vi "XYZ Ultrasonic Scanning Software 1.3.vi"() -> ()   [LabVIEW 2020]
doc: "The latest version of the ultrasonic scanning rig software."
uses:
  <instrlib>/Arcus Ethernet Driver 1.0.0/ArcusEthernetComm/classes/Controller/_Controller.lvclass
  <instrlib>/LeCroy Wave Series/LeCroy Wave Series.lvlib
panel:
  in  "stop":bool
  in  "Tab Control":T1(tab)
  in  "Check Osc Connection":bool
  out "Succesful Osc Connection":bool=TRUE
  in  "Check Rig Connection":bool
  out "Succesful Rig Connection":bool=TRUE
  in  "Error In":errorcluster
  in  "VISA Resource Name (Osc. Model Used)":refnum<visa-resource-name>
  in  "Move Y Distance":dbl
  in  "Set Starting Position":bool
  in  "Z Direction":bool=TRUE
  in  "Y Direction":bool=TRUE
  in  "Move X Distance":dbl
  in  "Move Z Distance":dbl
  in  "X Direction":bool=TRUE
  in  "Return To Home":bool
  in  "Move":bool
  in  "File Format":T2(radio)
  in  "File Name":string
  in  "Folder to Save A-Scan":path
  in  "Start A-Scan":bool
  in  "VISA resource name":refnum<visa-resource-name>
  in  "Source (0: Channel 1)":u16(ring) items=["Channel 1", "Channel 2", "Channel 3", "Channel 4", "Memory 1", "Memory 2", "Memory 3", "Memory 4", "Function 1", "Function 2", "Function 3", "Function 4", "Function 5", "Function 6", "Function 7", "Function 8"]
  out "A-Scan":waveform(dbl)(graph)
  in  "File Name for B-Scan":string
  in  "Folder to Save B-Scan":path
  in  "Folder to Save A-Scans":path
  in  "File Name for A-Scans":string
  in  "File Format":T2(radio)
  in  "Osc. Model":refnum<visa-resource-name>
  in  "Channel":u16(ring) items=["Channel 1", "Channel 2", "Channel 3", "Channel 4", "Memory 1", "Memory 2", "Memory 3", "Memory 4", "Function 1", "Function 2", "Function 3", "Function 4", "Function 5", "Function 6", "Function 7", "Function 8"]
  in  "Start B-Scan":bool
  in  "Initial X Direction":bool=TRUE
  in  "Initial Y Direction":bool=TRUE
  in  "Initial Z Direction":bool=TRUE
  in  "Confirm Scanning Parameters B-Scan":bool
  in  "Height (mm)":dbl
  in  "Width (mm)":dbl
  in  "Length (mm)":dbl
  in  "Select Axis To Scan":enum32{"No Selection", "X", "Y", "Z"}(radio)
  out "B-Scan":dbl[][](graph)
  in  "Folder to Save C-Scan":path
  in  "File Name for C-Scan":string
  in  "Source (0: Channel 1)":u16(ring) items=["Channel 1", "Channel 2", "Channel 3", "Channel 4", "Memory 1", "Memory 2", "Memory 3", "Memory 4", "Function 1", "Function 2", "Function 3", "Function 4", "Function 5", "Function 6", "Function 7", "Function 8"]
  in  "VISA resource name":refnum<visa-resource-name>
  in  "C-Scan Build Up Quantity":T3(radio)
  out "C-Scan":dbl[][](graph)
  in  "Scan C-Scan":bool
  in  "Length (mm)":dbl
  in  "Width (mm)":dbl
  in  "Height (mm)":dbl
  in  "?":bool
  in  "Initial X Direction":bool=TRUE
  in  "Initial Y Direction":bool=TRUE
  in  "Initial Z Direction":bool=TRUE
  in  "Select Plane To Scan":enum32{"No Selection", "XY", "XZ", "YZ"}(radio)
  in  "Folder to Save A-Scans":path
  in  "File Name for A-Scans":string
  in  "File Format":T2(radio)
  # "Moving To Starting Point (mm)"
  # "Scanning Tank Axes"
  # "Y"
  # "X"
  # "Z"
  # "Home ->"
  # "*Note - See user manual for scanning rig orientation to ensure correct axis directions"
  # "Scanning Parameters"
  # "Saving Parameters"
  # "Scanning Rig Parameters"
  # "Tank Dimensions"
  # "Y - Width"
  # "X - Length"
  # "Z - Height"
  # "Oscilloscope Parameters"
  # "Saving Parameters"
  # "*Note - See user manual for scanning rig orientation to ensure correct axis directions"
  # "Scanning Rig Parameters"
  # "Tank Dimensions"
  # "Y - Width"
  # "X - Length"
  # "Z - Height"
  # "Oscilloscope Parameters"
  # "Saving Parameters"
  # "*Note - See user manual for scanning rig orientation to ensure correct axis directions"
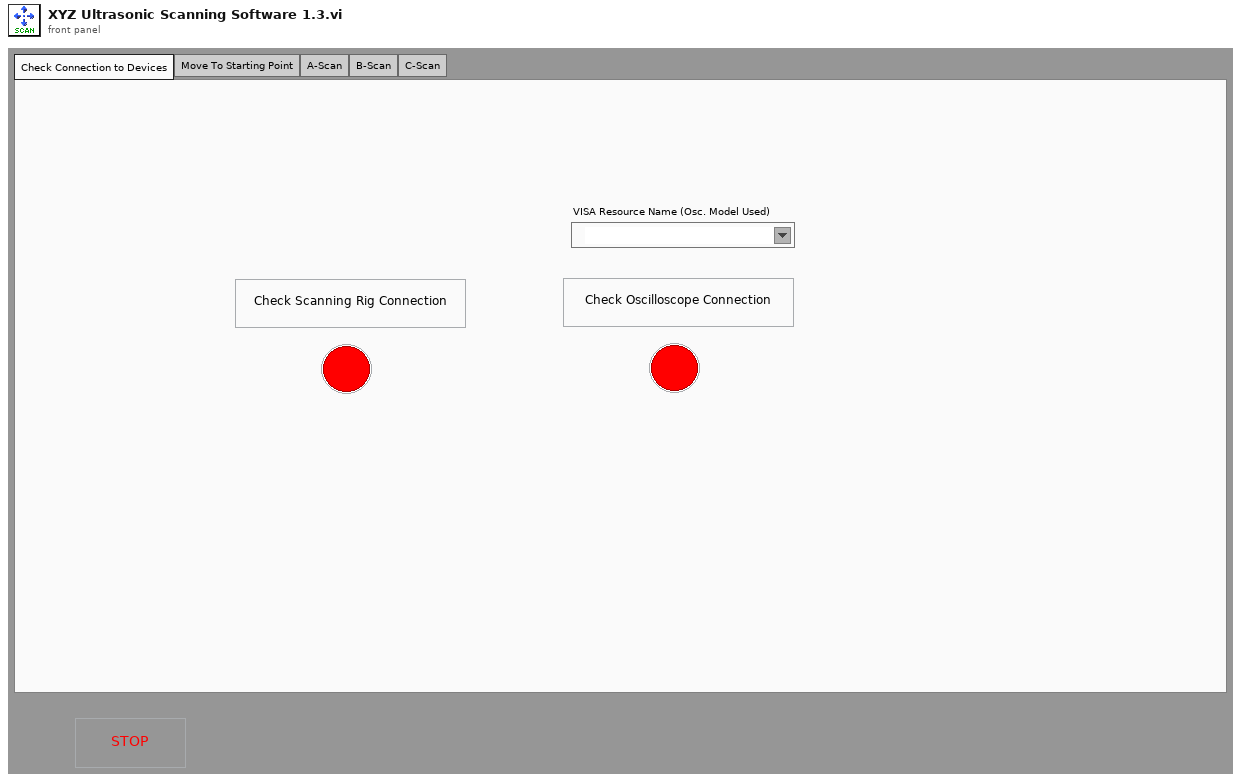
[diagram p1: front panel]
types:
  T1 = enum32{"Check Connection to Devices", "Move To Starting Point", "A-Scan", "B-Scan", "C-Scan"}
  T2 = enum32{"No Selection", "Do Not Save", "ASCII", "CSV", "MATLAB"}
  T3 = enum32{"No Selection", "Peak Positive", "Peak Negative", "Peak Magnitude", "Energy"}
  T4 = enum8{"Enabled", "Disabled", "Disabled and Grayed Out"}
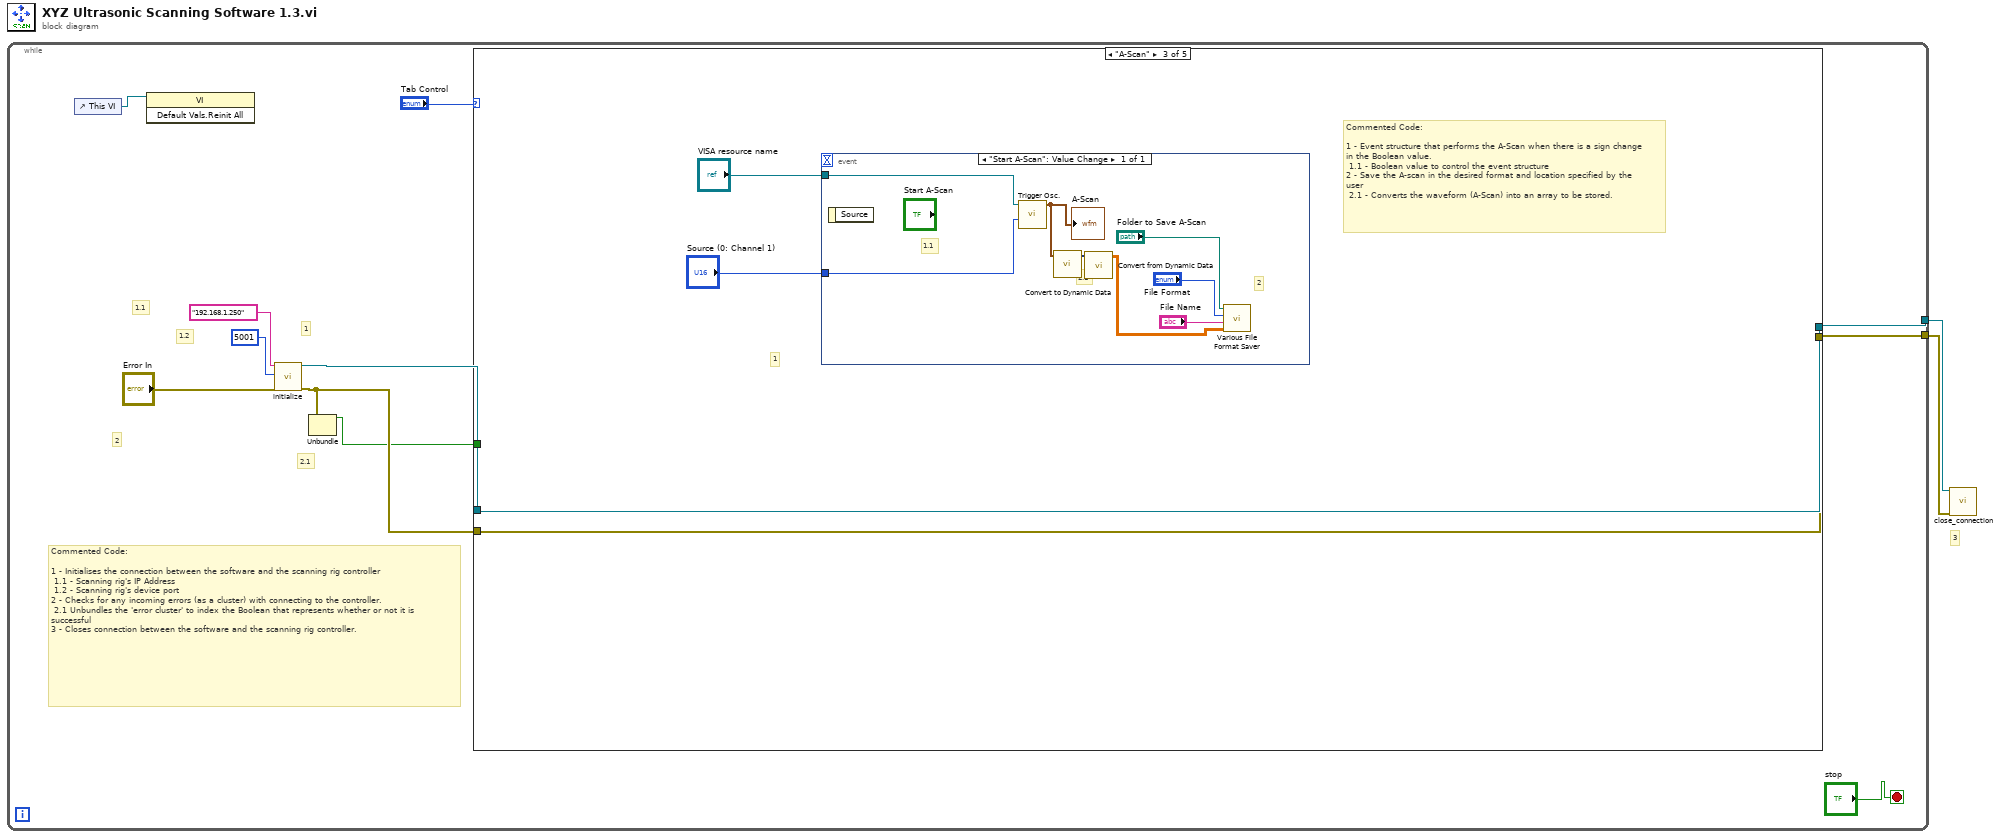
[diagram p0: block diagram]
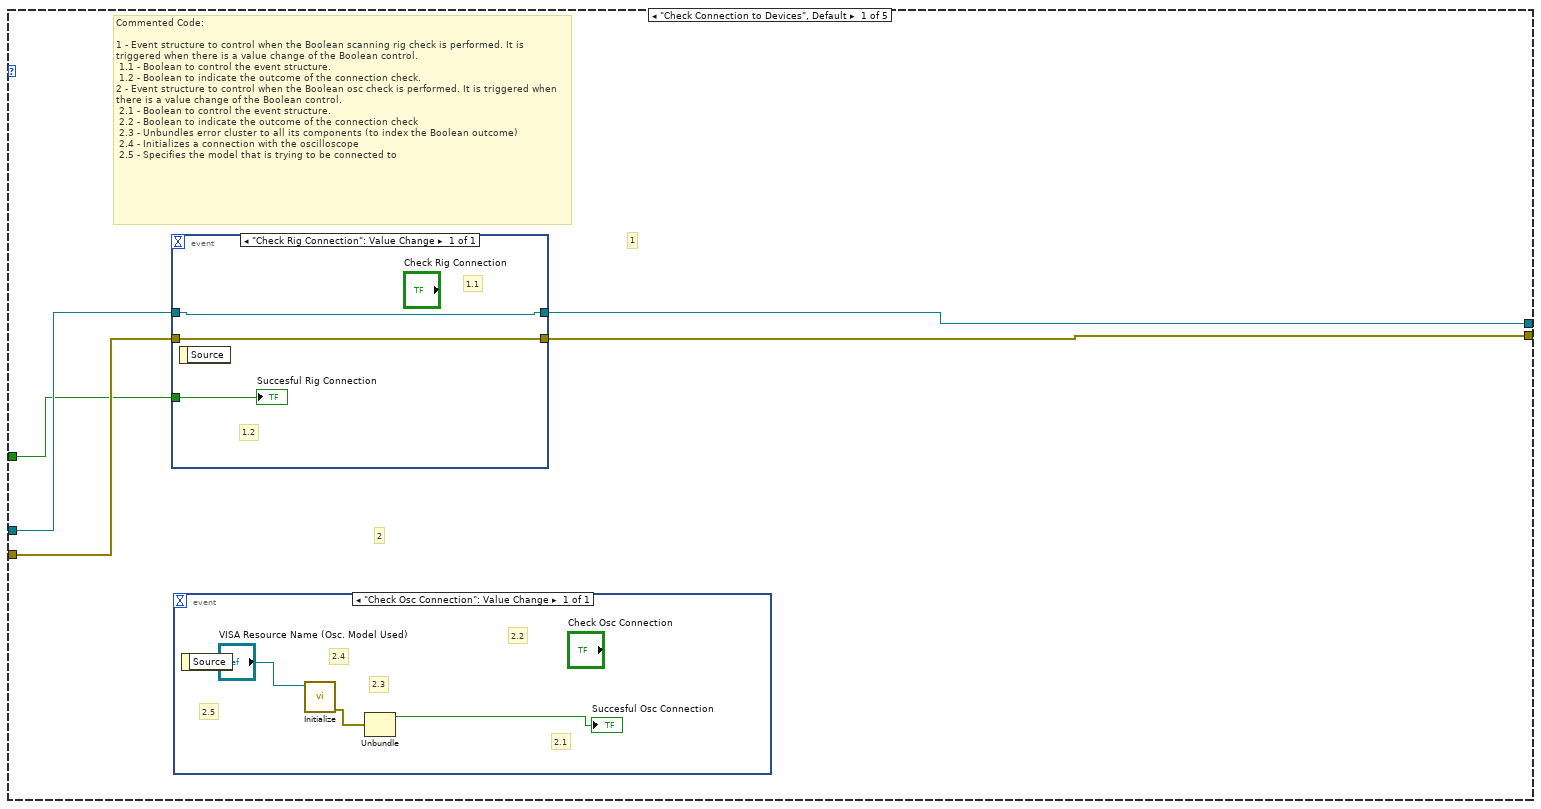
[diagram p2: hidden frame]
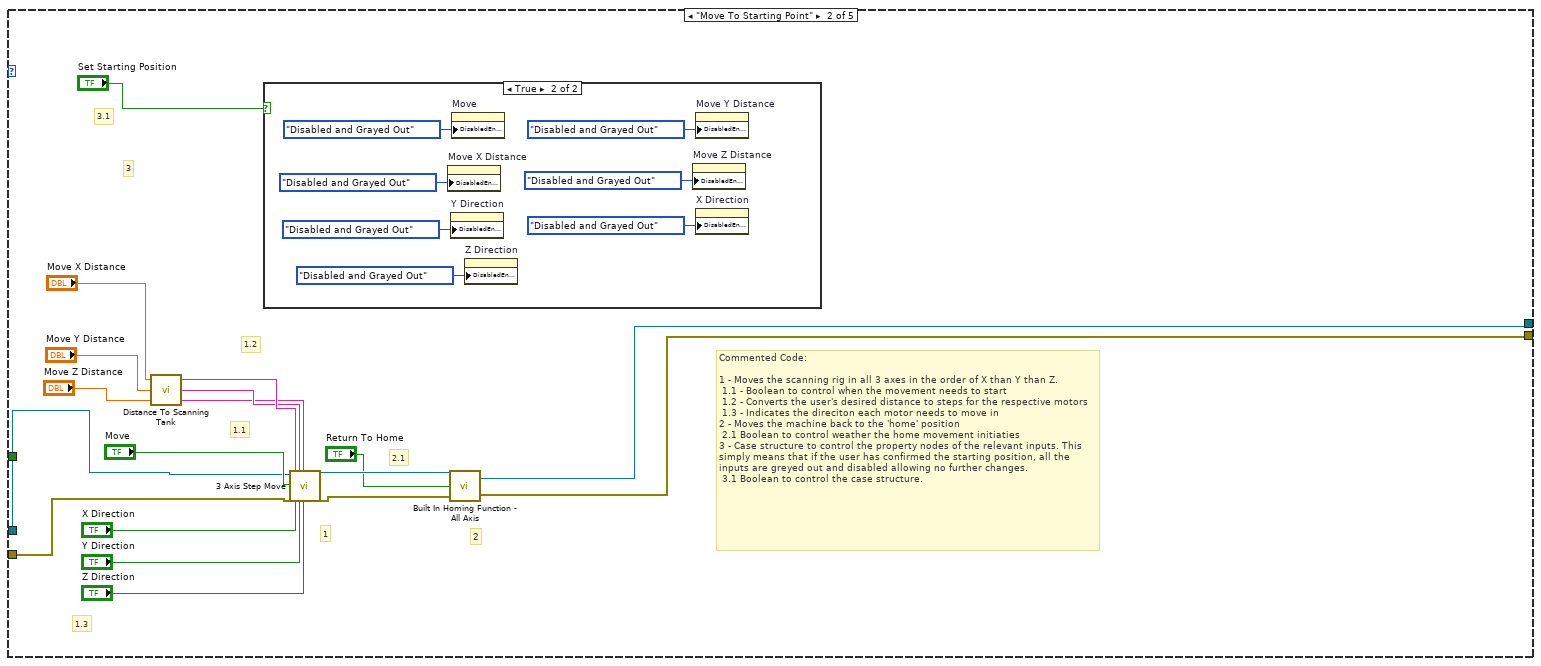
[diagram p3: hidden frame]
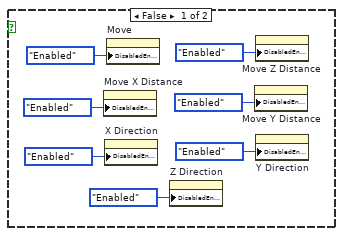
[diagram p4: hidden frame]
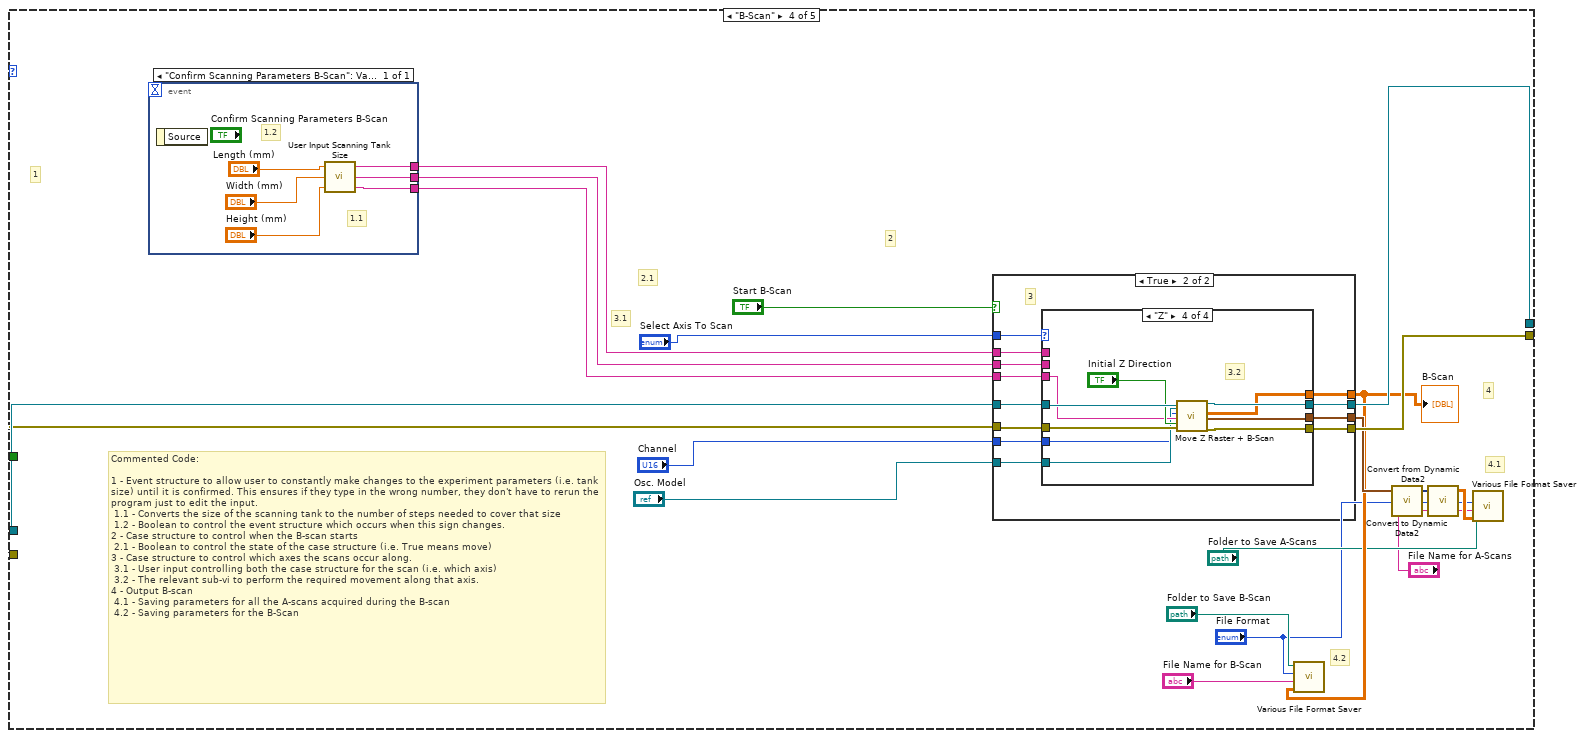
[diagram p5: hidden frame]
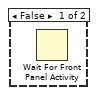
[diagram p6: hidden frame]
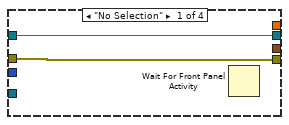
[diagram p7: hidden frame]
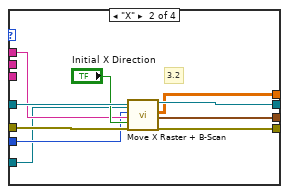
[diagram p8: hidden frame]
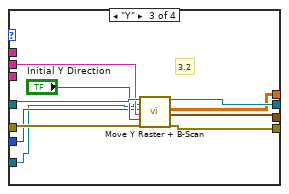
[diagram p9: hidden frame]
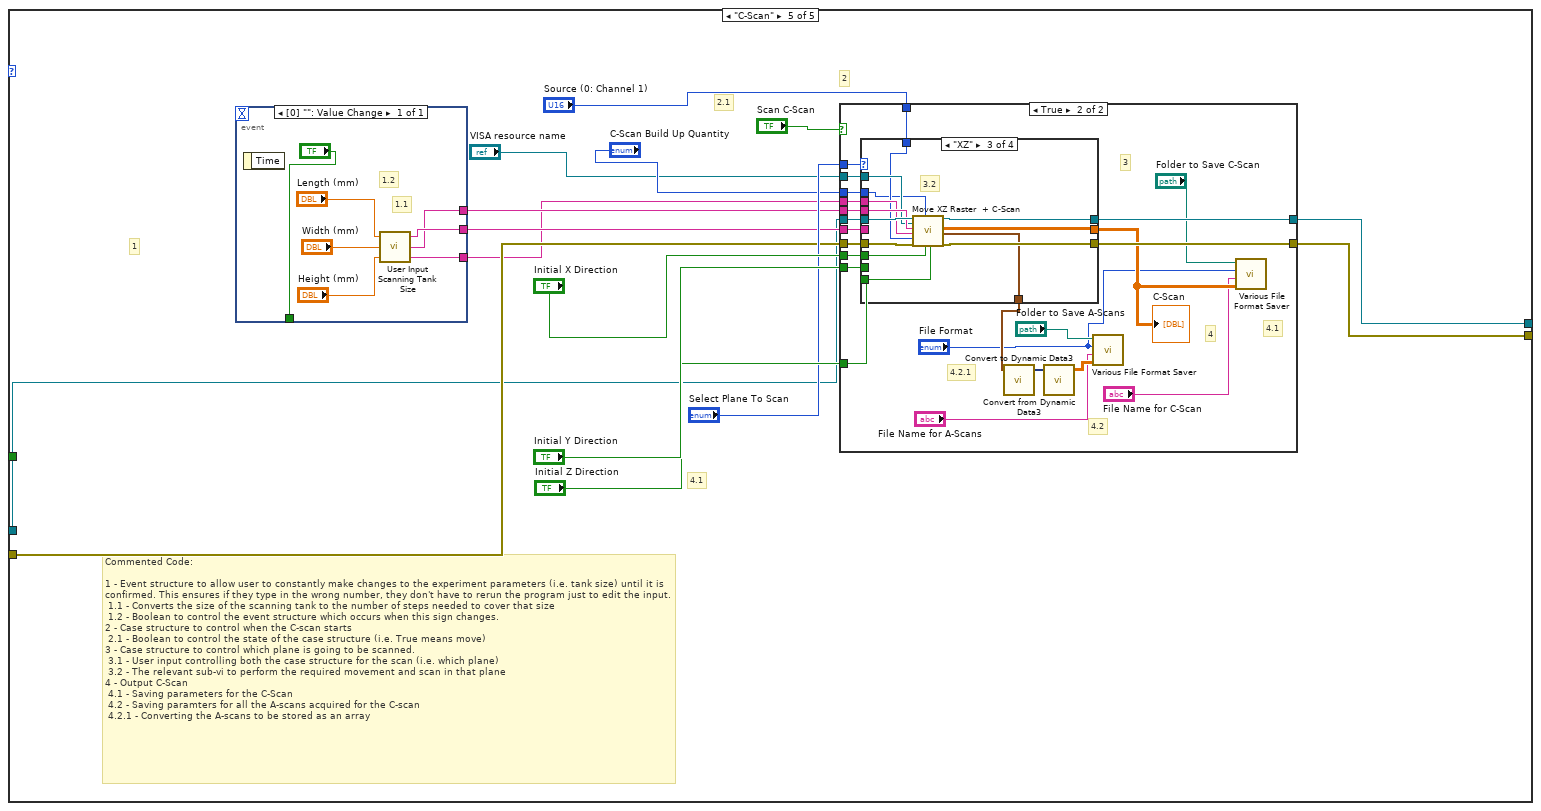
[diagram p10: hidden frame]
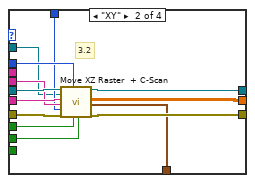
[diagram p13: hidden frame]
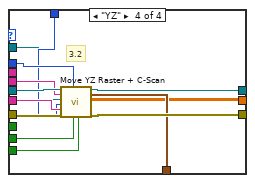
[diagram p14: hidden frame]
diagram:
  # "3"
  n1 = while {
    tunnel: [w6] -> w1
    tunnel: [w5] -> w2
    stop <- "stop" stop-if-true
    # "2"
    # "2.1"
    # "1.2"
    # "1.1"
    # "1"
    # "Commented Code:\n\n1 - Initialises the connection between the software and the scanning rig controller\n 1.1 - Scanning rig's IP Address\n 1.2 - Scanning rig's device port\n2 - Checks for any incoming errors (as a cluster) with connecting to the controller.  \n 2.1 Unbundles the 'error cluster' to index the Boolean that represents whether or not it is successful\n3 - Closes connection between the software and the scanning rig controller."
    n2 = control-ref of="This VI"() -> (w4:refnum<vi>)
    n3 = invoke class="VI" method="Default Vals.Reinit All"(reference=w4) -> ()  [unwired: 2 in, 3 out]
    n4 = call <instrlib>:"initialize.vi"("ip_address (in)"="192.168.1.250", "dev_port(def=5001)"=u16 5001, "error in (no error)"="Error In") -> ("reference (out)"=w12:refnum<class "_Controller.lvclass">, "error out"=w13:errorcluster)  [unwired: 15 in]
    n5 = Unbundle(w13) -> ("status"=w7:bool)  [unwired: 2 out]
    n6 = case shown="\"A-Scan\"" "Tab Control" {
      tunnel: w12 -> [w18 w32 w60 w88 w142]
      tunnel: [w16 w27 w60 w83 w150] -> w6
      tunnel: [w15 w28 w59 w81 w149] -> w5
      tunnel: w13 -> [w17 w31 w59 w87 w146]
      tunnel: w7 -> [w14 _ _ _ _]
      frame "Check Connection to Devices", Default {
        # "2"
        # "1"
        # "Commented Code:\n\n1 - Event structure to control when the Boolean scanning rig check is performed. It is triggered when there is a value change of the Boolean control. \n 1.1 - Boolean to control the event structure. \n 1.2 - Boolean to indicate the outcome of the connection check.\n2 - Event structure to control when the Boolean osc check is performed. It is triggered when there is a value change of the Boolean control. \n 2.1 - Boolean to control the event structure.\n 2.2 - Boolean to indicate the outcome of the connection check\n 2.3 - Unbundles error cluster to all its components (to index the Boolean outcome)\n 2.4 - Initializes a connection with the oscilloscope\n 2.5 - Specifies the model that is trying to be connected to"
        n7 = event shown="[0] \"Check Rig Connection\": Value Change" {
          selector: _ -> [_]
          dyn-events: _ -> [_]
          timeout: _ -> [_]
          tunnel: w18 -> [w24]
          tunnel: w17 -> [w23]
          tunnel: [w24] -> w16
          tunnel: [w23] -> w15
          tunnel: w14 -> [w22]
          event "Check Rig Connection": Value Change {
            # "1.1"
            # "1.2"
            n8 = event-data() -> ()  [unwired: 1 in, 1 out]
            "Succesful Rig Connection" <- w22
          }
        }
        n9 = event shown="[0] \"Check Osc Connection\": Value Change" {
          selector: _ -> [_]
          dyn-events: _ -> [_]
          timeout: _ -> [_]
          event "Check Osc Connection": Value Change {
            # "2.5"
            # "2.4"
            # "2.3"
            # "2.2"
            # "2.1"
            n10 = event-data() -> ()  [unwired: 1 in, 1 out]
            n11 = call <instrlib>:"Initialize.vi"("VISA resource name"="VISA Resource Name (Osc. Model Used)") -> ("error out"=w19:errorcluster)  [unwired: 9 in, 1 out]
            n12 = Unbundle(w19) -> ("status"=→"Succesful Osc Connection":bool)  [unwired: 2 out]
          }
        }
      }
      frame "Move To Starting Point" {
        # "3.1"
        # "3"
        # "2.1"
        # "2"
        # "1.3"
        # "1.1"
        # "1"
        # "1.2"
        # "Commented Code:\n\n1 - Moves the scanning rig in all 3 axes in the order of X than Y than Z.\n 1.1 - Boolean to control when the movement needs to start\n 1.2 - Converts the user's desired distance to steps for the respective motors\n 1.3 - Indicates the direciton each motor needs to move in\n2 - Moves the machine back to the 'home' position\n 2.1 Boolean to control weather the home movement initiaties \n3 - Case structure to control the property nodes of the relevant inputs. This simply means that if the user has confirmed the starting position, all the inputs are greyed out and disabled allowing no further changes.\n 3.1 Boolean to control the case structure."
        n13 = call "Distance To Scanning Tank.vi"("Move Z Distance (mm)"="Move Z Distance", "Move Y Distance (mm)"="Move Y Distance", "Move X Distance (mm)"="Move X Distance") -> ("Z Steps"=w40:string, "Y Steps"=w41:string, "X Steps"=w42:string)
        n14 = case shown="True" "Set Starting Position" {
          frame False {
            n15 = property on="Move X Distance" class="DigNum (strict)"("DisabledEnum"=T4."Enabled" ("Disabled")) -> ()  [unwired: 2 in, 2 out]
            n16 = property on="X Direction" class="Bool (strict)"("DisabledEnum"=T4."Enabled" ("Disabled")) -> ()  [unwired: 2 in, 2 out]
            n17 = property on="Move" class="Bool (strict)"("DisabledEnum"=T4."Enabled" ("Disabled")) -> ()  [unwired: 2 in, 2 out]
            n18 = property on="Z Direction" class="Bool (strict)"("DisabledEnum"=T4."Enabled" ("Disabled")) -> ()  [unwired: 2 in, 2 out]
            n19 = property on="Move Y Distance" class="DigNum (strict)"("DisabledEnum"=T4."Enabled" ("Disabled")) -> ()  [unwired: 2 in, 2 out]
            n20 = property on="Move Z Distance" class="DigNum (strict)"("DisabledEnum"=T4."Enabled" ("Disabled")) -> ()  [unwired: 2 in, 2 out]
            n21 = property on="Y Direction" class="Bool (strict)"("DisabledEnum"=T4."Enabled" ("Disabled")) -> ()  [unwired: 2 in, 2 out]
          }
          frame True {
            n22 = property on="Move X Distance" class="DigNum (strict)"("DisabledEnum"=T4."Disabled and Grayed Out" ("Disabled")) -> ()  [unwired: 2 in, 2 out]
            n23 = property on="Y Direction" class="Bool (strict)"("DisabledEnum"=T4."Disabled and Grayed Out" ("Disabled")) -> ()  [unwired: 2 in, 2 out]
            n24 = property on="Move" class="Bool (strict)"("DisabledEnum"=T4."Disabled and Grayed Out" ("Disabled")) -> ()  [unwired: 2 in, 2 out]
            n25 = property on="Z Direction" class="Bool (strict)"("DisabledEnum"=T4."Disabled and Grayed Out" ("Disabled")) -> ()  [unwired: 2 in, 2 out]
            n26 = property on="Move Z Distance" class="DigNum (strict)"("DisabledEnum"=T4."Disabled and Grayed Out" ("Disabled")) -> ()  [unwired: 2 in, 2 out]
            n27 = property on="Move Y Distance" class="DigNum (strict)"("DisabledEnum"=T4."Disabled and Grayed Out" ("Disabled")) -> ()  [unwired: 2 in, 2 out]
            n28 = property on="X Direction" class="Bool (strict)"("DisabledEnum"=T4."Disabled and Grayed Out" ("Disabled")) -> ()  [unwired: 2 in, 2 out]
          }
        }
        n29 = call "3 Axis Step Move.vi"("Reference In"=w32, "Move"="Move", "Error In"=w31, "X Steps"=w42, "Direction X"="X Direction", "Y Steps"=w41, "Direction Y"="Y Direction", "Z Steps"=w40, "Direcition Z"="Z Direction") -> ("Reference Out"=w30:refnum<class "_Controller.lvclass">, "Error Out"=w26:errorcluster)  [unwired: 17 in]
        n30 = call "Built In Homing Function - All Axis.vi"("Error In"=w26, "Home"="Return To Home", "Reference In"=w30) -> ("Error Out"=w28:errorcluster, "Reference Out"=w27:refnum<class "_Controller.lvclass">)
      }
      frame "A-Scan" {
        # "1"
        # "Commented Code:\n\n1 - Event structure that performs the A-Scan when there is a sign change in the Boolean value.\n 1.1 - Boolean value to control the event structure\n2 - Save the A-scan in the desired format and location specified by the user\n 2.1 - Converts the waveform (A-Scan) into an array to be stored."
        n31 = event shown="[0] \"Start A-Scan\": Value Change" {
          selector: _ -> [_]
          dyn-events: _ -> [_]
          timeout: _ -> [_]
          tunnel: "VISA resource name" -> [w68]
          tunnel: "Source (0: Channel 1)" -> [w67]
          event "Start A-Scan": Value Change {
            # "2"
            # "2.1"
            # "1.1"
            n32 = event-data() -> ()  [unwired: 1 in, 1 out]
            n33 = call "Trigger Osc..vi"("Source (0: Channel 1)"=w67, "VISA resource name"=w68) -> ("Waveform Data"=w66:waveform(dbl))  [unwired: 9 in]
            "A-Scan" <- w66
            n34 = call "Convert to Dynamic Data"("Waveform"=w66) -> ("Dynamic Data Type"=w65:dynamicdata)  [unwired: 3 in]
            n35 = call "Convert from Dynamic Data"("Dynamic Data Type"=w65) -> ("Array"=w61:dbl[][])  [unwired: 3 in]
            n36 = call "Various File Format Saver.vi"("Incoming Data to be Saved"=w61, "File Name"="File Name", "File Format"="File Format", "Folder to Save Data"="Folder to Save A-Scan") -> ()  [unwired: 8 in]
          }
        }
      }
      frame "B-Scan" {
        # "4.2"
        # "4.1"
        # "4"
        # "3.1"
        # "2.1"
        # "2"
        # "1"
        # "Commented Code:\n\n1 - Event structure to allow user to constantly make changes to the experiment parameters (i.e. tank size) until it is confirmed. This ensures if they type in the wrong number, they don't have to rerun the program just to edit the input.\n 1.1 - Converts the size of the scanning tank to the number of steps needed to cover that size\n 1.2 - Boolean to control the event structure which occurs when this sign changes.\n2 - Case structure to control when the B-scan starts\n 2.1 - Boolean to control the state of the case structure (i.e. True means move) \n3 - Case structure to control which axes the scans occur along. \n 3.1 - User input controlling both the case structure for the scan (i.e. which axis)\n 3.2 - The relevant sub-vi to perform the required movement along that axis. \n4 - Output B-scan\n 4.1 - Saving parameters for all the A-scans acquired during the B-scan\n 4.2 - Saving parameters for the B-Scan"
        n37 = event shown="[0] \"Confirm Scanning Parameters B-Scan\": Value Change" {
          selector: _ -> [_]
          dyn-events: _ -> [_]
          timeout: _ -> [_]
          tunnel: [w135] -> w84
          tunnel: [w134] -> w85
          tunnel: [w133] -> w86
          event "Confirm Scanning Parameters B-Scan": Value Change {
            # "1.2"
            # "1.1"
            n38 = event-data() -> ()  [unwired: 1 in, 1 out]
            n39 = call "User Input Scanning Tank Size.vi"("Height (mm)"="Height (mm)", "Width (mm)"="Width (mm)", "Length (mm)"="Length (mm)") -> ("Z Steps"=w135:string, "Y Steps"=w134:string, "X Steps"=w133:string)
          }
        }
        n40 = case shown="True" "Start B-Scan" {
          tunnel: "Select Axis To Scan" -> [_ w100]
          tunnel: w88 -> [_ w99]
          tunnel: w87 -> [_ w93]
          tunnel: w86 -> [_ w98]
          tunnel: w85 -> [_ w97]
          tunnel: w84 -> [_ w96]
          tunnel: [_ w95] -> w81
          tunnel: [_ w94] -> w83
          tunnel: [_ w92] -> w77
          tunnel: [_ w91] -> w74
          tunnel: "Osc. Model" -> [_ w90]
          tunnel: "Channel" -> [_ w89]
          frame False {
            n41 = Wait For Front Panel Activity() -> ()  [unwired: 3 in, 1 out]
          }
          frame True {
            # "3"
            n42 = case shown="\"Z\"" w100 {
              tunnel: w99 -> [w102 w112 w122 w132]
              tunnel: w93 -> [w101 w109 w121 w131]
              tunnel: [w101 w107 w117 w127] -> w95
              tunnel: w98 -> [_ w110 _ _]
              tunnel: w97 -> [_ _ w119 _]
              tunnel: w96 -> [_ _ _ w129]
              tunnel: [w102 w108 w118 w128] -> w94
              tunnel: [_ w106 w116 w126] -> w92
              tunnel: [_ w105 w115 w125] -> w91
              tunnel: w90 -> [_ w103 w113 w124]
              tunnel: w89 -> [_ w104 w114 w123]
              frame "No Selection" {
                n43 = Wait For Front Panel Activity() -> ()  [unwired: 3 in, 1 out]
              }
              frame "X" {
                # "3.2"
                n44 = call "Move X Raster + B-Scan.vi"("Reference In"=w112, "VISA resource name"=w103, "Source (0: Channel 1)"=w104, "X Number of Steps"=w110, "Initial Direction"="Initial X Direction", "Error In"=w109) -> ("Reference Out"=w108:refnum<class "_Controller.lvclass">, "B-Scan"=w105:dbl[][], "A-Scan"=w106:waveform(dbl)[], "Error Out"=w107:errorcluster)  [unwired: 10 in]
              }
              frame "Y" {
                # "3.2"
                n45 = call "Move Y Raster + B-Scan.vi"("Reference In"=w122, "VISA resource name"=w113, "Source (0: Channel 1)"=w114, "Y Number of Steps"=w119, "Initial Direction"="Initial Y Direction", "Error In"=w121) -> ("Reference Out"=w118:refnum<class "_Controller.lvclass">, "B-Scan"=w115:dbl[][], "A-Scan"=w116:waveform(dbl)[], "Error Out"=w117:errorcluster)  [unwired: 10 in]
              }
              frame "Z" {
                # "3.2"
                n46 = call "Move Z Raster + B-Scan.vi"("Reference In"=w132, "VISA resource name"=w124, "Source (0: Channel 1)"=w123, "Z Number of Steps"=w129, "Initial Direction"="Initial Z Direction", "Error In"=w131) -> ("Reference Out"=w128:refnum<class "_Controller.lvclass">, "B-Scan"=w125:dbl[][], "A-Scan"=w126:waveform(dbl)[], "Error Out"=w127:errorcluster)  [unwired: 10 in]
              }
            }
          }
        }
        "B-Scan" <- w74
        n47 = call "Various File Format Saver.vi"("Incoming Data to be Saved"=w74, "File Name"="File Name for B-Scan", "File Format"="File Format", "Folder to Save Data"="Folder to Save B-Scan") -> ()  [unwired: 8 in]
        n48 = call "Convert to Dynamic Data2"("Array of Waveforms"=w77) -> ("Dynamic Data Type"=w76:dynamicdata)  [unwired: 3 in]
        n49 = call "Convert from Dynamic Data2"("Dynamic Data Type"=w76) -> ("Array"=w75:dbl[][])  [unwired: 3 in]
        n50 = call "Various File Format Saver.vi"("Incoming Data to be Saved"=w75, "File Name"="File Name for A-Scans", "File Format"="File Format", "Folder to Save Data"="Folder to Save A-Scans") -> ()  [unwired: 8 in]
      }
      frame "C-Scan" {
        # "4.1"
        # "2.1"
        # "2"
        # "1"
        # "Commented Code:\n\n1 - Event structure to allow user to constantly make changes to the experiment parameters (i.e. tank size) until it is confirmed. This ensures if they type in the wrong number, they don't have to rerun the program just to edit the input.\n 1.1 - Converts the size of the scanning tank to the number of steps needed to cover that size\n 1.2 - Boolean to control the event structure which occurs when this sign changes.\n2 - Case structure to control when the C-scan starts\n 2.1 - Boolean to control the state of the case structure (i.e. True means move) \n3 - Case structure to control which plane is going to be scanned. \n 3.1 - User input controlling both the case structure for the scan (i.e. which plane)\n 3.2 - The relevant sub-vi to perform the required movement and scan in that plane\n4 - Output C-Scan\n 4.1 - Saving parameters for the C-Scan\n 4.2 - Saving paramters for all the A-scans acquired for the C-scan\n 4.2.1 - Converting the A-scans to be stored as an array"
        n51 = event shown="[0] \"\": Value Change" {
          selector: _ -> [_]
          dyn-events: _ -> [_]
          timeout: _ -> [_]
          tunnel: [w219] -> w145
          tunnel: [w218] -> w144
          tunnel: [w217] -> w143
          tunnel: ["?"] -> _
          event Value Change {
            # "1.1"
            # "1.2"
            n52 = event-data() -> ()  [unwired: 1 in, 1 out]
            n53 = call "User Input Scanning Tank Size.vi"("Height (mm)"="Height (mm)", "Width (mm)"="Width (mm)", "Length (mm)"="Length (mm)") -> ("Z Steps"=w217:string, "Y Steps"=w218:string, "X Steps"=w219:string)
          }
        }
        n54 = case shown="True" "Scan C-Scan" {
          tunnel: "Select Plane To Scan" -> [_ w176]
          tunnel: "Initial X Direction" -> [_ w175]
          tunnel: "Initial Y Direction" -> [_ w174]
          tunnel: "Initial Z Direction" -> [_ w173]
          tunnel: w142 -> [_ w172]
          tunnel: w146 -> [_ w171]
          tunnel: [_ w170] -> w150
          tunnel: [_ w169] -> w149
          tunnel: w145 -> [_ w168]
          tunnel: w144 -> [_ w167]
          tunnel: w143 -> [_ w166]
          tunnel: "C-Scan Build Up Quantity" -> [_ w165]
          tunnel: "Source (0: Channel 1)" -> [_ w164]
          tunnel: "VISA resource name" -> [_ w163]
          frame False {
          }
          frame True {
            # "4.2.1"
            # "4.2"
            # "4.1"
            # "4"
            # "3"
            n55 = case shown="\"XZ\"" w176 {
              tunnel: w175 -> [_ w185 w199 _]
              tunnel: w174 -> [_ w184 _ w208]
              tunnel: w173 -> [_ _ w198 w207]
              tunnel: w172 -> [_ w189 w200 w215]
              tunnel: w171 -> [_ w188 w201 w209]
              tunnel: [_ w187 w190 w214] -> w170
              tunnel: [_ w186 w202 w213] -> w169
              tunnel: w168 -> [_ w183 _ w211]
              tunnel: w167 -> [_ w182 w197 w212]
              tunnel: w166 -> [_ _ w196 _]
              tunnel: [_ w177 w195 w210] -> w159
              tunnel: w165 -> [_ w181 w191 w205]
              tunnel: [_ w180 w194 w206] -> w162
              tunnel: w164 -> [_ w179 w192 w204]
              tunnel: w163 -> [_ w178 w193 w203]
              frame "No Selection", Default {
              }
              frame "XY" {
                # "3.2"
                n56 = call "Move XZ Raster  + C-Scan.vi"("Reference In"=w189, "VISA resource name"=w178, "X Number of Steps"=w183, "Z Number of Steps"=w182, "Source (0: Channel 1)"=w179, "Error In"=w188, "C-Scan Build Up Quantity"=w181, "Initial X Direction"=w185, "Initial Z Direction"=w184) -> ("Reference Out"=w187:refnum<class "_Controller.lvclass">, "C-Scan"=w180:dbl[][], "A-Scan (for C-Scan)"=w177:waveform(dbl)[], "Error Out"=w186:errorcluster)  [unwired: 7 in]
              }
              frame "XZ" {
                # "3.2"
                n57 = call "Move XZ Raster  + C-Scan.vi"("Reference In"=w200, "VISA resource name"=w193, "X Number of Steps"=w197, "Z Number of Steps"=w196, "Source (0: Channel 1)"=w192, "Error In"=w201, "C-Scan Build Up Quantity"=w191, "Initial X Direction"=w199, "Initial Z Direction"=w198) -> ("Reference Out"=w190:refnum<class "_Controller.lvclass">, "C-Scan"=w194:dbl[][], "A-Scan (for C-Scan)"=w195:waveform(dbl)[], "Error Out"=w202:errorcluster)  [unwired: 7 in]
              }
              frame "YZ" {
                # "3.2"
                n58 = call "Move YZ Raster + C-Scan.vi"("Reference In"=w215, "Y Number of Steps"=w212, "VISA resource name"=w203, "Source (0: Channel 1)"=w204, "Z Number of Steps"=w211, "Error In"=w209, "C-Scan Build Up Quantity"=w205, "Initial Y Direction"=w208, "Initial Z Direction"=w207) -> ("Reference Out"=w214:refnum<class "_Controller.lvclass">, "A-Scan (for C-Scan)"=w210:waveform(dbl)[], "C-Scan"=w206:dbl[][], "Error Out"=w213:errorcluster)  [unwired: 7 in]
              }
            }
            "C-Scan" <- w162
            n59 = call "Convert to Dynamic Data3"("Array of Waveforms"=w159) -> ("Dynamic Data Type"=w161:dynamicdata)  [unwired: 3 in]
            n60 = call "Convert from Dynamic Data3"("Dynamic Data Type"=w161) -> ("Array"=w160:dbl[][])  [unwired: 3 in]
            n61 = call "Various File Format Saver.vi"("Incoming Data to be Saved"=w160, "File Name"="File Name for A-Scans", "File Format"="File Format", "Folder to Save Data"="Folder to Save A-Scans") -> ()  [unwired: 8 in]
            n62 = call "Various File Format Saver.vi"("Incoming Data to be Saved"=w162, "File Name"="File Name for C-Scan", "File Format"="File Format", "Folder to Save Data"="Folder to Save C-Scan") -> ()  [unwired: 8 in]
          }
        }
      }
    }
  }
  n63 = call <instrlib>:"close_connection.vi"("reference (in)"=w1, "error in (no error)"=w2) -> ()  [unwired: 16 in, 2 out]
